vi "AB_860_900_Project_Build_Info.vi"(7 "action":T1, 8 "error in (no error)":errorcluster, 10 "buildInfo in":T2, 11 "Object In":T3) -> (0 "error out":errorcluster, 2 "buildInfo out":T2, 3 "Object Out":T3)   [LabVIEW 2020]
uses:
  <resource>/Framework/Providers/API/ItemRef.ctl
  <vilib>/AppBuilder/RW_Project/AB_RW_Project_PropBag_Action.ctl
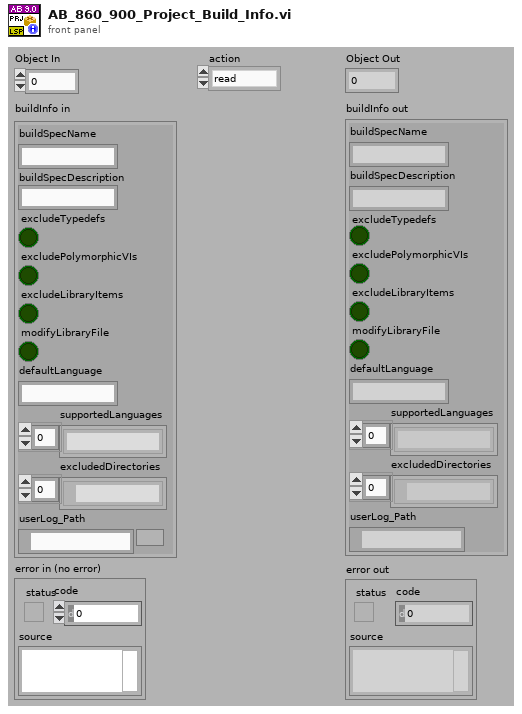
[diagram p1: front panel]
types:
  T1 = typedef "AB_RW_Project_PropBag_Action.ctl" = enum16{"read", "write", "clear", "readPrevious", "writePrevious", "clearPrevious"}
  T2 = cluster{"buildSpecName":string, "buildSpecDescription":string, "excludeTypedefs":bool, "excludePolymorphicVIs":bool, "excludeLibraryItems":bool, "modifyLibraryFile":bool, "defaultLanguage":string, "supportedLanguages":string[], "excludedDirectories":path[], "userLog_Path":path}
  T3 = typedef "ItemRef.ctl" = u64
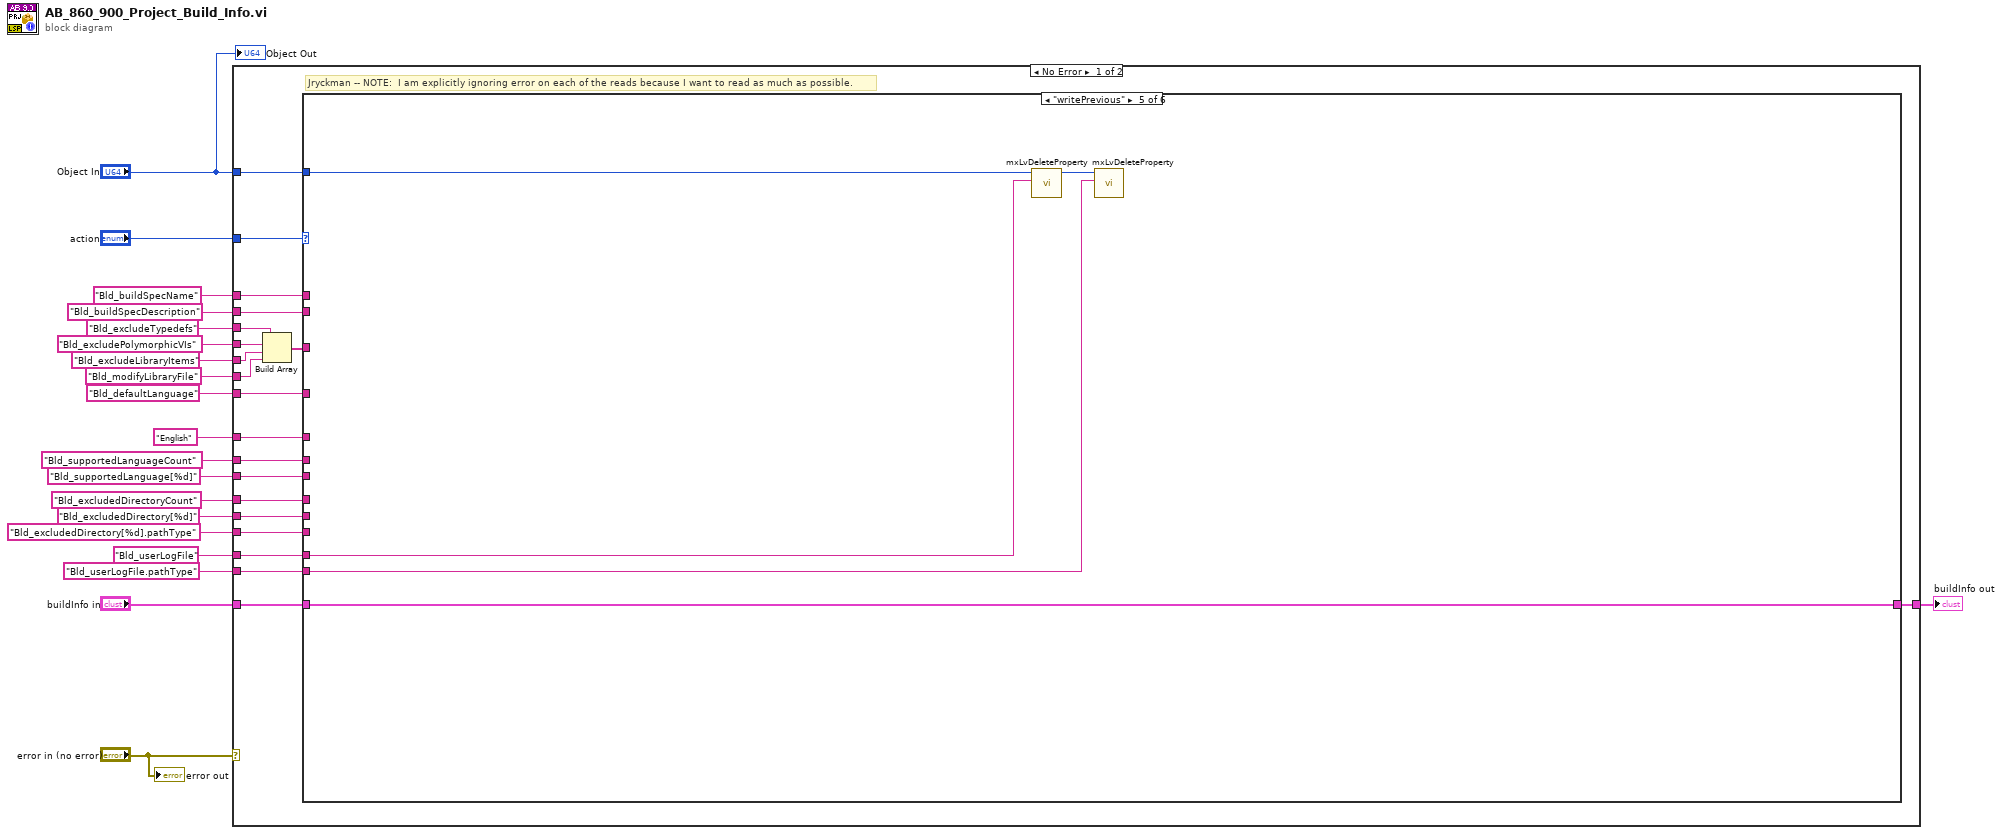
[diagram p0: block diagram]
diagram:
  n1 = case shown="No Error" "error in (no error)" {
    tunnel: "Object In" -> [w40 _]
    tunnel: [w29 _] -> w18
    tunnel: "Bld_buildSpecDescription" ("Tag") -> [w39 _]
    tunnel: "Bld_excludeTypedefs" ("Tag") -> [w25 _]
    tunnel: "Bld_defaultLanguage" ("Tag") -> [w38 _]
    tunnel: "English" ("Tag") -> [w37 _]
    tunnel: "Bld_supportedLanguageCount" ("Tag") -> [w36 _]
    tunnel: "Bld_supportedLanguage[%d]" ("Tag") -> [w35 _]
    tunnel: "Bld_excludedDirectoryCount" ("Tag") -> [w34 _]
    tunnel: "Bld_excludedDirectory[%d]" ("Tag") -> [w33 _]
    tunnel: "Bld_excludedDirectory[%d].pathType" ("Tag") -> [w32 _]
    tunnel: "buildInfo in" -> [w31 _]
    tunnel: "action" -> [w30 _]
    tunnel: "Bld_excludePolymorphicVIs" ("Tag") -> [w28 _]
    tunnel: "Bld_excludeLibraryItems" ("Tag") -> [w27 _]
    tunnel: "Bld_modifyLibraryFile" ("Tag") -> [w26 _]
    tunnel: "Bld_buildSpecName" ("Tag") -> [w23 _]
    tunnel: "Bld_userLogFile" ("Tag") -> [w22 _]
    tunnel: "Bld_userLogFile.pathType" ("Tag") -> [w21 _]
    frame No Error {
      # "Jryckman -- NOTE:  I am explicitly ignoring error on each of the reads because I want to read as much as possible."
      n2 = Build Array(w25, w28, w27, w26) -> (w24:string[])
      n3 = case shown="\"writePrevious\"" w30 {
        tunnel: w40 -> [_ _ _ _ w48 _]
        tunnel: w39 -> [_ _ _ _ _ _]
        tunnel: w38 -> [_ _ _ _ _ _]
        tunnel: w37 -> [_ _ _ _ _ _]
        tunnel: w36 -> [_ _ _ _ _ _]
        tunnel: w35 -> [_ _ _ _ _ _]
        tunnel: w34 -> [_ _ _ _ _ _]
        tunnel: w33 -> [_ _ _ _ _ _]
        tunnel: w32 -> [_ _ _ _ _ _]
        tunnel: w31 -> [w41 w42 w43 w44 w49 w50]
        tunnel: [w41 w42 w43 w44 w49 w50] -> w29
        tunnel: w24 -> [_ _ _ _ _ _]
        tunnel: w23 -> [_ _ _ _ _ _]
        tunnel: w22 -> [_ _ _ _ w47 _]
        tunnel: w21 -> [_ _ _ _ w45 _]
        frame "read" {
        }
        frame "write" {
        }
        frame "clear" {
        }
        frame "readPrevious" {
        }
        frame "writePrevious" {
          n4 = call <resource>:"mxLvDeleteProperty.vi"("Tag"=w47, "Item"=w48) -> ("Item"=w46:T3)  [unwired: 1 in, 8 out]
          n5 = call <resource>:"mxLvDeleteProperty.vi"("Tag"=w45, "Item"=w46) -> ()  [unwired: 1 in, 9 out]
        }
        frame "clearPrevious" {
        }
      }
    }
    frame Error {
    }
  }
  "buildInfo out" <- w18
  "Object Out" <- "Object In"
  "error out" <- "error in (no error)"
